vi "Core Destroy.vi"(8 "error in (no error)":errorcluster, 11 "CIFTemplateNode in":refnum<class "CIFCorePlugin.lvclass">) -> (0 "error out":errorcluster, 3 "CIFTemplateNode out":refnum<class "CIFCorePlugin.lvclass">)   [LabVIEW 2021, in "CIFCorePlugin.lvclass"]
uses:
  CIFCorePlugin.lvclass
  Grpc/CIFCorePlugin_server/RPC Service/PluginCore/PluginCore.lvclass
  Channels/CIFChannelMng/CIFChannelMng.lvclass
  <vilib>/gRPC/LabVIEW gRPC Servicer/ServiceBase/ServiceBase.lvclass
  <vilib>/CIF Foundation/CIF CIPC/CIF_NI_CIPC.lvlib
  C:/Program Files/National Instruments/LabVIEW 2021/vi.lib/gRPC/LabVIEW gRPC Servicer/ServiceBase/ServiceBase.lvclass
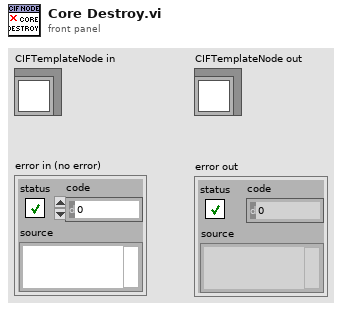
[diagram p1: front panel]
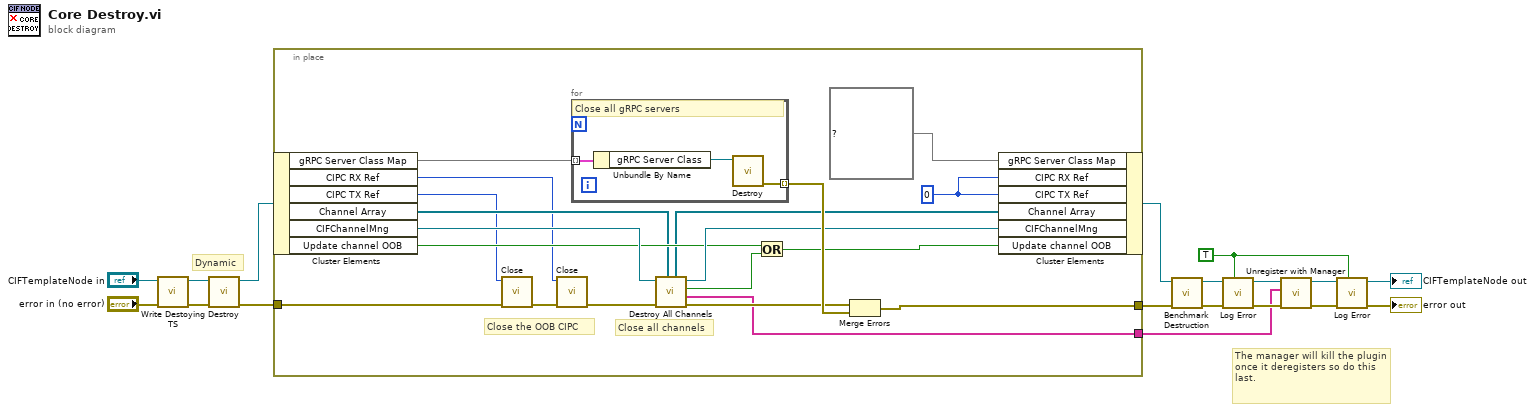
[diagram p0: block diagram]
diagram:
  w3 = TRUE ("Write to Terminal")
  # "The manager will kill the plugin once it deregisters so do this last."
  # "Dynamic"
  n1 = call "Write Destoying TS.vi"("error in (no error)"="error in (no error)", "CIFCorePlugin in"="CIFTemplateNode in") -> ("error out"=w13:errorcluster, "CIFCorePlugin out"=w14:refnum<class "CIFCorePlugin.lvclass">)  [unwired: 8 in]
  n2 = call-dynamic "Destroy.vi"("error in (no error)"=w13, "CIFTemplateNode in"=w14) -> ("error out"=w11:errorcluster, "CIFTemplateNode out"=w12:refnum<class "CIFCorePlugin.lvclass">)  [unwired: 8 in]
  n3 = in-place {
    in-place-border: w11 -> [w24]
    in-place-border: [w35] -> w10
    in-place-border: [w25] -> w1
    w19 = u64 0 ("CIPC RX Ref")
    # "Close all channels"
    # "Close the OOB CIPC"
    n4 = in-place-cluster #1(w12) -> ("gRPC Server Class Map"=w37:map{string, refnum<class "ServiceBase.lvclass">}, "CIPC RX Ref"=w22:u64, "CIPC TX Ref"=w23:u64, "Channel Array"=w26:refnum<class "CIFChannels.lvclass">[], "CIFChannelMng"=w32:refnum<class "CIFChannelMng.lvclass">, "Update channel OOB"=w30:bool)
    n5 = call <vilib>:"Close.vi"("error in (no error)"=w24, "CIPC Reference"=w23) -> ("error out"=w21:errorcluster)  [unwired: 9 in]
    n6 = call <vilib>:"Close.vi"("error in (no error)"=w21, "CIPC Reference"=w22) -> ("error out"=w20:errorcluster)  [unwired: 9 in]
    n7 = for {
      tunnel: w37 -> [w40] mode=indexing
      tunnel: [w38] -> w36 mode=indexing
      # "Close all gRPC servers"
      n8 = Unbundle By Name(w40) -> ("gRPC Server Class"=w39:refnum<class "ServiceBase.lvclass">)
      n9 = call-dynamic "Destroy.vi"("SignalGeneratorService in"=w39) -> ("error out"=w38:errorcluster)  [unwired: 9 in, 1 out]
    }
    n10 = call "Destroy All Channels.vi"("Channel Array in"=w26, "error in (no error)"=w20, "CIFChannelMng in"=w32) -> ("error out"=w33:errorcluster, "Unregister Channels"=w25:string[], "Update Channel OOB"=w29:bool, "CIFChannelMng out"=w31:refnum<class "CIFChannelMng.lvclass">, "Channel Array out"=w27:refnum<class "CIFChannels.lvclass">[])  [unwired: 4 in]
    n11 = Or(x=w30, y=w29) -> (x .or. y?=w28:bool)
    n12 = Merge Errors(w33, w36) -> (w35:errorcluster)
    n13 = in-place-cluster #1("gRPC Server Class Map"=map{string, refnum<class "PluginCore.lvclass">} {}, "CIPC RX Ref"=w19, "CIPC TX Ref"=w19, "Channel Array"=w27, "CIFChannelMng"=w31, "Update channel OOB"=w28) -> (w2:refnum<class "CIFCorePlugin.lvclass">)
  }
  n14 = call "Benchmark Destruction.vi"("error in (no error)"=w10, "CIFCorePlugin in"=w2) -> ("error out"=w15:errorcluster, "CIFCorePlugin out"=w16:refnum<class "CIFCorePlugin.lvclass">)  [unwired: 8 in]
  n15 = call "Log Error.vi"("Write to Terminal"=w3, "error in (no error)"=w15, "CIFCorePlugin in"=w16) -> ("error out"=w9:errorcluster, "CIFCorePlugin out"=w8:refnum<class "CIFCorePlugin.lvclass">)  [unwired: 7 in]
  n16 = call "Unregister with Manager.vi"("error in (no error)"=w9, "Unregister Channels"=w1, "CIFCorePlugin in"=w8) -> ("error out"=w6:errorcluster, "CIFCorePlugin out"=w7:refnum<class "CIFCorePlugin.lvclass">)  [unwired: 7 in]
  n17 = call "Log Error.vi"("Write to Terminal"=w3, "error in (no error)"=w6, "CIFCorePlugin in"=w7) -> ("error out"=→"error out":errorcluster, "CIFCorePlugin out"=→"CIFTemplateNode out":refnum<class "CIFCorePlugin.lvclass">)  [unwired: 7 in]
